vi "Read Saved Ringdowns.vi"() -> ()   [LabVIEW 2014]
uses:
  <vilib>/Platform/TimedLoop/XDataNode/timing_clust.ctl
  <vilib>/Platform/TimedLoop/XDataNode/nitl_modes.ctl
  <vilib>/Platform/TimedLoop/XDataNode/wakeup.ctl
  <vilib>/Platform/TimedLoop/XDataNode/XDataNode.xnode
  <vilib>/Platform/TimedLoop/XDataNode/XDNodeRunTimeDep.lvlib
  Reusable/General/Math Utilities.lvlib
  <vilib>/Analysis/NI_AALBase.lvlib
panel:
  out "size(s) 2":i32[](array[numeric])
  in  "Data":i32
  out "Waveform Graph 3":i16[][](graph)
  out "appended array":timestamp[](array[timestamp]) format="%<%H:%M:%S%2u>T"
  out "error out":errorcluster
  out "Waveform Chart":cluster{"mean":dbl, "mean":dbl}(graph)
  out "size(s)":i32[](array[numeric])
  out "Waveform Graph 2":dbl[](graph)
  in  "index (row)":i32
  out "Waveform Graph":dbl[][](graph)
  out "Numeric":i32
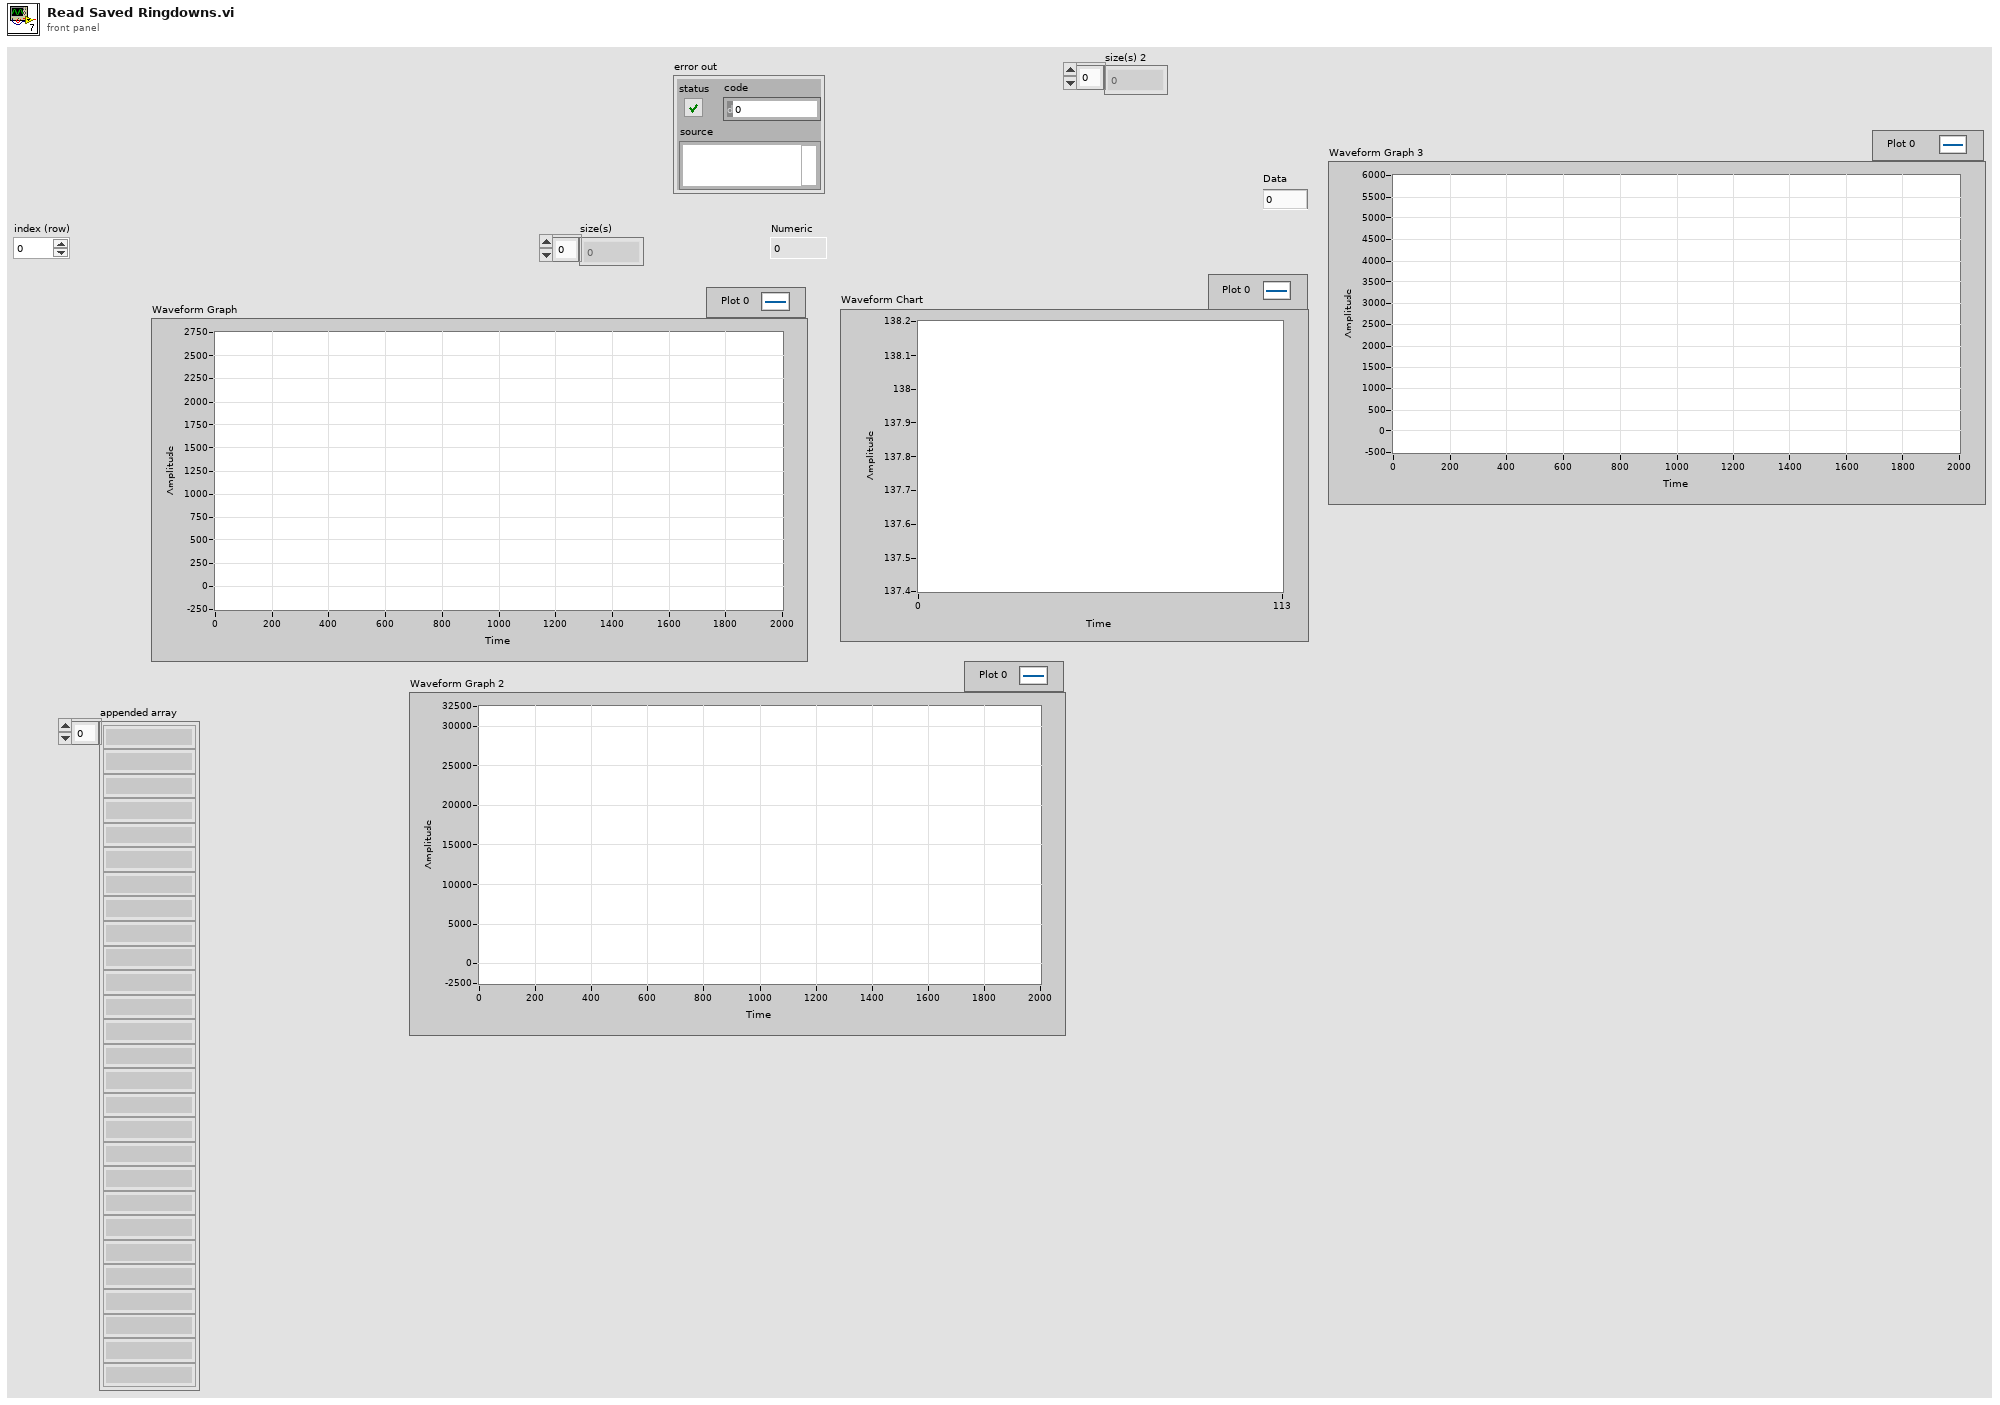
[diagram p1: front panel]
types:
  T1 = typedef "XDNodeRunTimeDep.lvlib/timing_clust.ctl" = cluster{"Expected End [f-1]":u64, "Actual End [f-1]":u64, "Finished Late? [f-1]":bool, "Expected End [i-1]":u64, "Actual End [i-1]":u64, "Finished Late? [i-1]":bool, "Expected Start [i]":u64, "Actual Start [i]":u64, "Expected Start [f]":u64, "Actual Start [f]":u64, "Source Name":string, "Structure Name":string, "Period":i64, "Deadline":i64, "Offset":i64, "Start":i64, "Priority":i32, "Timeout":i32, "Mode":T2, "Wakeup Reason":T3, "Error":errorcluster, "Source Type":string, "Secondary Source Type":string, "Global End Time":u64, "Global Start Time":u64, "Frame Duration":u64, "Iteration Duration":u64, "Assigned CPU":i32, "I/O Scan Engine Mode":u32}
  T2 = typedef "XDNodeRunTimeDep.lvlib/nitl_modes.ctl" = enum32{"No Change", "Process missed periods, maintain original phase", "Discard missed periods, maintain original phase", "Process missed periods, ignore original phase", "Discard missed periods, ignore original phase"}
  T3 = typedef "XDNodeRunTimeDep.lvlib/wakeup.ctl" = enum32{"Normal", "Aborted", "Asynchronous wakeup", "Timing source error", "Timed loop error", "Timeout"}
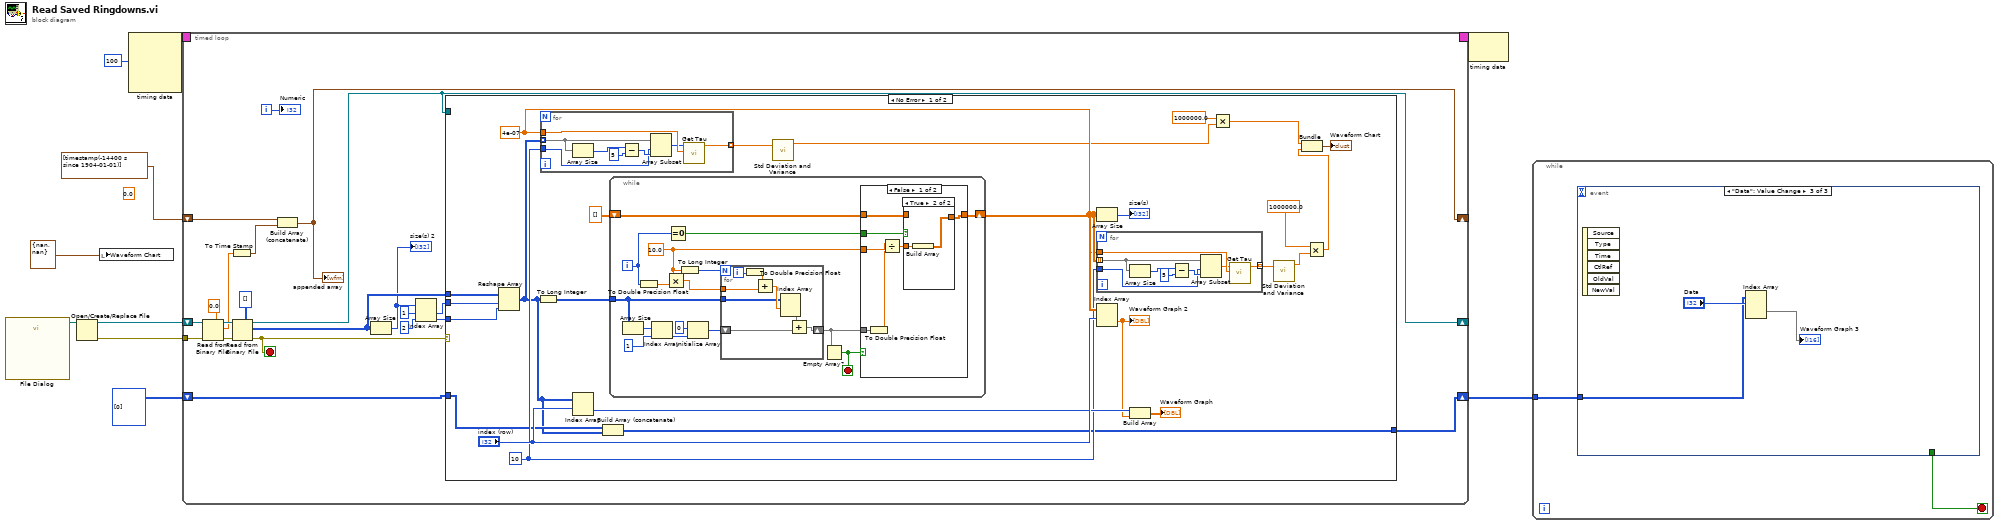
[diagram p0: block diagram]
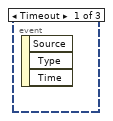
[diagram p2: hidden frame]
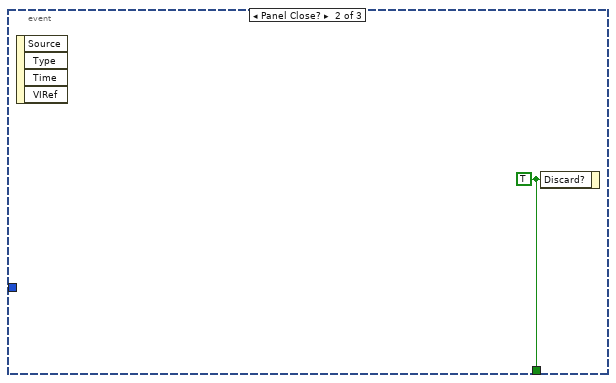
[diagram p3: hidden frame]
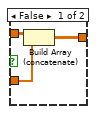
[diagram p4: hidden frame]
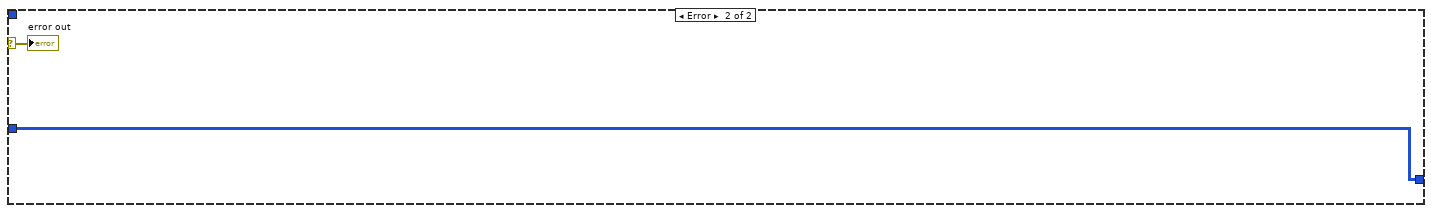
[diagram p6: hidden frame]
diagram:
  (unwired) 0.0 ("data")
  n1 = call "File Dialog"() -> ("selected path"=w5:path)  [unwired: 12 in, 3 out]
  n2 = Open/Create/Replace File(file path (use dialog)=w5) -> (refnum out=w10:refnum<file>, error out=w6:errorcluster)  [unwired: 5 in, 1 out]
  n3 = local write "Waveform Chart"(cluster{"mean":dbl, "mean":dbl} {"mean"=nan, "mean"=nan} ("Waveform Chart")) -> ()
  n4 = node-c288(i64 100 ("Period")) -> (w9:T1)  [unwired: 3 in]
  n5 = timed-loop {
    shift-right: [w22] -> _
    shift-left: w10 -> [w21]
    timing: w9 -> [_]
    timing-out: [_] -> w8
    tunnel: w6 -> [w20]
    shift-right: [w13] -> _
    shift-left: timestamp[] [timestamp(-14400 s since 1904-01-01)] -> [w15]
    shift-right: [w11] -> w1
    shift-left: i16[][][] [[[0]]] ("output array") -> [w12]
    i -> [w29]
    stop <- w30 stop-if-true
    n6 = Read from Binary File(5:0.0, 8:w20, 11:w21) -> (0:w18:errorcluster, 2:w16:dbl, 3:w19:refnum<file>)  [unwired: 3 in, 1 out]
    n7 = To Time Stamp(1:w16) -> (0:w14:timestamp)
    n8 = Read from Binary File(5:i16[][][] [], 8:w18, 11:w19) -> (0:w30:errorcluster, 2:w28:i16[][][], 3:w22:refnum<file>)  [unwired: 3 in, 1 out]
    n9 = Build Array (concatenate)(w15, w14) -> (w13:timestamp[])
    "appended array" <- w13
    n10 = Array Size(array=w28) -> (size(s)=w27:i32[])
    "size(s) 2" <- w27
    n11 = Index Array(array=w27, index #1=1 ("index"), index #2=2 ("index")) -> (element #1=w24:i32, element #2=w23:i32)
    n12 = case shown="No Error" w30 {
      selector: w30 -> [_ w111]
      tunnel: w28 -> [w56 _]
      tunnel: w24 -> [w55 _]
      tunnel: w23 -> [w54 _]
      tunnel: w22 -> [_ _]
      tunnel: w12 -> [w34 w110]
      tunnel: [w32 w110] -> w11
      frame No Error {
        w41 = 10 ("index")
        w42 = 4e-07 ("Dt")
        n13 = Reshape Array(w56, w55, w54) -> (w33:i16[][])
        n14 = To Long Integer(number=w33) -> (32bit integer=w51:i32[][])
        n15 = for {
          tunnel: w33 -> [w70] mode=indexing
          tunnel: [w72] -> w45 mode=indexing
          tunnel: w42 -> [w71]
          tunnel: w41 -> [w65]
          n16 = Array Size(array=w70) -> (size(s)=w69:i32)
          n17 = Subtract(x=w69, y=5) -> (x-y=w66:i32)
          n18 = Array Subset(array=w70, index=w65, length=w66) -> (w67:i16[])
          n19 = call "Get Tau.vi"("Dt"=w71, "X"=w67) -> ("tau"=w72:dbl)  [unwired: 6 in, 3 out]
        }
        n20 = Index Array(array=w33, index (row)="index (row)") -> (element=w49:i16[])  [unwired: 1 in]
        n21 = Build Array (concatenate)(w34, w33) -> (w32:i16[][][])
        n22 = while {
          tunnel: w51 -> [w84]
          shift-right: [w77] -> w46
          shift-left: dbl[][] [] ("output array") -> [w86]
          i -> [w74]
          stop <- w88 stop-if-true
          w75 = 10.0 ("x")
          n23 = Array Size(array=w84) -> (size(s)=w83:i32[])
          n24 = To Double Precision Float(number=w74) -> (double precision float=w73:dbl)
          n25 = Index Array(array=w83, index=1) -> (element=w81:i32)
          n26 = Multiply(x=w75, y=w73) -> (x*y=w85:dbl)
          n27 = Equal To 0?(x=w74) -> (x = 0?=w87:bool)
          n28 = To Long Integer(number=w75) -> (32bit integer=w76:i32)
          n29 = Initialize Array(0 ("element"), w81) -> (w79:i32[])
          n30 = for {
            N: w76 -> [_]
            tunnel: w84 -> [w95]
            tunnel: w85 -> [w91]
            shift-right: [w92] -> w78
            shift-left: w79 -> [w93]
            i -> [w89]
            n31 = To Double Precision Float(number=w89) -> (double precision float=w90:dbl)
            n32 = Add(x=w90, y=w91) -> (x+y=w96:dbl)
            n33 = Index Array(array=w95, index (row)=w96) -> (element=w94:i32[])  [unwired: 1 in]
            n34 = Add(x=w94, y=w93) -> (x+y=w92:i32[])
          }
          n35 = Empty Array?(array=w78) -> (empty?=w88:bool)
          n36 = case shown="False" w88 {
            tunnel: w87 -> [w103 _]
            tunnel: [w102 w109] -> w77
            tunnel: w86 -> [w101 w109]
            tunnel: w78 -> [w98 _]
            tunnel: w75 -> [w99 _]
            frame False {
              n37 = To Double Precision Float(number=w98) -> (double precision float=w97:dbl[])
              n38 = Divide(x=w97, y=w99) -> (x/y=w100:dbl[])
              n39 = case shown="True" w103 {
                tunnel: [w105 w108] -> w102
                tunnel: w101 -> [w106 _]
                tunnel: w100 -> [w104 w107]
                frame False {
                  n40 = Build Array (concatenate)(w106, w104) -> (w105:dbl[][])
                }
                frame True {
                  n41 = Build Array(w107) -> (w108:dbl[][])
                }
              }
            }
            frame True {
            }
          }
        }
        n42 = call <vilib>:"Std Deviation and Variance.vi"("X"=w45) -> ("mean"=w36:dbl)  [unwired: 1 in, 2 out]
        n43 = Array Size(array=w46) -> (size(s)=→"size(s)":i32[])
        n44 = for {
          tunnel: w46 -> [w61] mode=indexing
          tunnel: [w64] -> w44 mode=indexing
          tunnel: w42 -> [w63]
          tunnel: w41 -> [w57]
          n45 = Array Size(array=w61) -> (size(s)=w60:i32)
          n46 = Subtract(x=w60, y=5) -> (x-y=w59:i32)
          n47 = Array Subset(array=w61, index=w57, length=w59) -> (w58:dbl[])
          n48 = call "Get Tau.vi"("Dt"=w63, "X"=w58) -> ("tau"=w64:dbl)  [unwired: 6 in, 3 out]
        }
        n49 = Index Array(array=w46, index (row)="index (row)") -> (element=w48:dbl[])  [unwired: 1 in]
        "Waveform Graph 2" <- w48
        n50 = Build Array(w49, w48) -> (→"Waveform Graph":dbl[][])
        n51 = Multiply(x=1000000.0, y=w36) -> (x*y=w35:dbl)
        n52 = call <vilib>:"Std Deviation and Variance.vi"("X"=w44) -> ("mean"=w40:dbl)  [unwired: 1 in, 2 out]
        n53 = Multiply(x=1000000.0, y=w40) -> (x*y=w38:dbl)
        n54 = Bundle(w35, w38) -> (→"Waveform Chart":cluster{dbl, dbl})  [unwired: 1 in]
      }
      frame Error {
        "error out" <- w111
      }
    }
    "Numeric" <- w29
  }
  n55 = node-c288(w8) -> ()  [unwired: 1 out]
  n56 = while {
    tunnel: w1 -> [w114]
    stop <- w115 stop-if-true
    n57 = event shown="[2] \"Data\": Value Change" {
      selector: _ -> [_ _ _]
      dyn-events: _ -> [_ _ _]
      timeout: _ -> [_ _ _]
      tunnel: [_ w116 _] -> w115
      tunnel: w114 -> [_ _ w118]
      event Timeout {
        n58 = event-data() -> ()  [unwired: 1 in, 3 out]
      }
      event Panel Close? {
        w116 = TRUE ("Discard?")
        n59 = event-data() -> ()  [unwired: 1 in, 4 out]
        n60 = event-data("Discard?"=w116) -> ()  [unwired: 1 in, 1 out]
      }
      event "Data": Value Change {
        n61 = event-data() -> ()  [unwired: 1 in, 6 out]
        n62 = Index Array(array=w118, index (dim 0)="Data") -> (element=→"Waveform Graph 3":i16[][])  [unwired: 2 in]
      }
    }
  }
